vi "UHR-Fleezers Control (host) -Leonardo 04-2018 V3.vi"(0 "Tab Control":T5(tab)=enum."Trap Control (RF)") -> ()   [LabVIEW 2013] (continued)
      event "Phase adj. (AI1)", "+ phase (AI1)", "- phase (AI1)": Value Change {
        n481 = event-data() -> ()  [unwired: 7 out]
        n482 = Negate(x="Phase adj. (AI1)") -> (-x=w846:i16)
        n483 = Select(t=w846, s="- phase (AI1)", f="Phase adj. (AI1)") -> (s? t:f=w845:i16)
        n484 = xnode "Read/Write Control"("FPGA VI Reference In"=w849, "error in"=w848, "Phase count adjustment"=w845) -> ("FPGA VI Reference Out"=w844:T20, "error out"=w843:errorcluster)
        n485 = Or(x="- phase (AI1)", y="+ phase (AI1)") -> (x .or. y?=w840:bool)
        n486 = xnode "Read/Write Control"("FPGA VI Reference In"=w844, "error in"=w843, "+ phase"=w840) -> ("error out"=w839:errorcluster)  [unwired: 1 out]
      }
      event "Signals to Plot": Double Click {
        w852 = u32 9868950 ("Color Box")
        n487 = event-data() -> ("Row"=w854:i32)  [unwired: 9 out]
        n488 = property on="All Signals" class="WFChart (strict)"("Active Plot"=w854) -> (error out=w865:errorcluster)  [unwired: 2 in, 1 out]
        n489 = property on="All Signals" class="WFChart (strict)" props=["Plot", "Visible?", "Plot", "Plot Color"](error in=w865) -> (error out=w864:errorcluster, "Plot.Visible?"=w863:bool)  [unwired: 1 in, 2 out]
        n490 = Select(t=FALSE ("Plot.Visible"), s=w863, f=TRUE ("Plot.Visible")) -> (s? t:f=w858:bool)
        n491 = property on="All Signals" class="WFChart (strict)"(error in=w864, "Plot.Visible?"=w858) -> (error out=w860:errorcluster)  [unwired: 1 in, 1 out]
        n492 = property on="All Signals" class="WFChart (strict)"(error in=w860) -> (error out=w855:errorcluster, "Plot.Plot Color"=w859:u32)  [unwired: 1 in, 1 out]
        n493 = property on="Signals to Plot" class="LstBox (strict)"(error in=w855, "Active Row"=w854) -> (error out=w853:errorcluster)  [unwired: 1 in, 1 out]
        n494 = Select(t=w859, s=w858, f=u32 0) -> (s? t:f=w856:u32)
        n495 = property on="Signals to Plot" class="LstBox (strict)"(error in=w853, "CellFontColor"=w856, "SelColor"=w852, "CellBG"=w852, "CellFontSize"=u32 20 ("Active Row:Cell Font:Size"), "CellFontBold"=TRUE ("Active Row:Cell Font:Bold")) -> ()  [unwired: 1 in, 2 out]
      }
      event "Dynamic Force FB": Value Change {
        n496 = event-data() -> ()  [unwired: 7 out]
        n497 = xnode "Read/Write Control"("FPGA VI Reference In"=w867, "Dynamic Force FB (Ronen)"="Dynamic Force FB") -> ()  [unwired: 1 in, 2 out]
      }
      event "BD 1 Frequency 1 (MHz)", "BD 1 Frequency 2 (MHz)", "BD 1 Frequency 3 (MHz)", "BD 2 Frequency 1 (MHz)", "BD 2 Frequency 2 (MHz)", "BD 2 Frequency 3 (MHz)", "Trap Delta (MHz)": Value Change {
        # "anytime one of the frequencies is changed, write it to the RF board UNLESS Set 2 is being oscillated. The oscillation\nscript writes the frequencies to the RF board."
        n498 = event-data() -> ("CtlRef"=w870:refnum<vi>)  [unwired: 6 out]
        n499 = control-ref of="Trap Delta (MHz)"() -> (w869:refnum<vi>)
        n500 = Equal?(x=w869, y=w870) -> (x = y?=w868:bool)
        n501 = case shown="False" "Oscillate Set 2" {
          tunnel: w873 -> [w894 _]
          tunnel: [w893 w906] -> w872
          tunnel: w871 -> [w892 w906]
          tunnel: w868 -> [w879 _]
          frame False {
            n502 = case shown="False" "Symmetric manual \ntrap motion" {
              tunnel: ["T2 for asymmetric\n(MHz)" w905] -> w880
              tunnel: "Trap Delta (MHz)" -> [w899 w904]
              tunnel: [w898 w901] -> w876
              frame False {
                n503 = Subtract(x="T2 for asymmetric\n(MHz)", y=w899) -> (x-y=w898:dbl)
              }
              frame True {
                n504 = Divide(x=w904, y=2) -> (x/y=w902:dbl)
                n505 = Subtract(x="Middle freq for \nsymmetric (MHz)", y=w902) -> (x-y=w901:dbl)
                n506 = Add(x="Middle freq for \nsymmetric (MHz)", y=w902) -> (x+y=w905:dbl)
              }
            }
            n507 = local read "BD 1 Frequency 2 (MHz)"() -> (w881:dbl)
            n508 = local write "BD 1 Frequency 1 (MHz)"(w876) -> ()
            n509 = Select(t=w880, s=w879, f=w881) -> (s? t:f=w878:dbl)
            n510 = local read "Y RF Frequency Limits (MHz)"() -> (w882:T16)
            n511 = local read "X RF Frequency Limits (MHz)"() -> (w883:T16)
            n512 = local read "BD 1 Frequency 3 (MHz)"() -> (w895:dbl)
            n513 = local write "BD 1 Frequency 2 (MHz)"(w878) -> ()
            n514 = local read "BD 2 Frequency 1 (MHz)"() -> (w886:dbl)
            n515 = local read "BD 2 Frequency 2 (MHz)"() -> (w885:dbl)
            n516 = local read "BD 2 Frequency 3 (MHz)"() -> (w896:dbl)
            n517 = call "set RF board frequency - interlace.vi"("Board 2 Frequency Limits"=w882, "Board 1 Frequency Limits"=w883, "error in"=w892, "FPGA VI Reference In"=w894, "Board 2 Frequency 3 (MHz)"=w896, "Board 1 Frequency 3 (MHz)"=w895, "Board 2 Frequency 2 (MHz)"=w885, "Board 2 Frequency 1 (MHz)"=w886, "Board 1 Frequency 2 (MHz)"=w878, "Board 1 Frequency 1  (MHz)"=w876) -> ("error out"=w893:errorcluster)  [unwired: 1 out]
            n518 = Subtract(x=w886, y=w885) -> (x-y=w890:dbl)
            n519 = Subtract(x=w878, y=w876) -> (x-y=w891:dbl)
            n520 = Square(x=w890) -> (x^2=w888:dbl)
            n521 = Square(x=w891) -> (x^2=w889:dbl)
            n522 = Add(x=w889, y=w888) -> (x+y=w887:dbl)
            n523 = Square Root(x=w887) -> (sqrt(x)=w884:dbl)
            n524 = local write "Trap Delta (MHz)"(w884) -> ()
            n525 = property on="Initial delta (MHz)" class="DigNum (strict)"("Val(Sgnl)"=w884) -> ()  [unwired: 2 in, 2 out]
          }
          frame True {
          }
        }
      }
      event "Round T1 X": Value Change {
        n526 = event-data() -> ()  [unwired: 7 out]
        n527 = local read "BD 1 Frequency 1 (MHz)"() -> (w909:dbl)
        n528 = Round To Nearest(number=w909) -> (nearest integer value=w908:dbl)
        n529 = property on="BD 1 Frequency 1 (MHz)" class="DigNum (strict)"("Val(Sgnl)"=w908) -> ()  [unwired: 2 in, 2 out]
      }
      event "Round T2 X": Value Change {
        n530 = event-data() -> ()  [unwired: 7 out]
        n531 = local read "BD 1 Frequency 2 (MHz)"() -> (w911:dbl)
        n532 = Round To Nearest(number=w911) -> (nearest integer value=w910:dbl)
        n533 = property on="BD 1 Frequency 2 (MHz)" class="DigNum (strict)"("Val(Sgnl)"=w910) -> ()  [unwired: 2 in, 2 out]
      }
      event "Stop All": Value Change {
        n534 = event-data() -> ()  [unwired: 7 out]
        n535 = call "hamilton_controller.vi"("action"=T21."DISCONNECT") -> ()  [unwired: 10 in, 1 out]
        n536 = local read "Stop All"() -> (w914:bool)
      }
      event "Delayed Interlace Start": Value Change {
        n537 = event-data() -> ()  [unwired: 7 out]
        n538 = flat-sequence {
          frame #0 {
            n539 = Multiply(x="Delay to Interlace (s)", y=1000.0) -> (x*y=w917:dbl)
            n540 = Wait (ms)(milliseconds to wait=w917) -> ()  [unwired: 1 out]
          }
          frame #1 {
            n541 = property on="Green laser mode" class="RadioBtnsControl (strict)"("Val(Sgnl)"=enum32{"Laser ON", "Laser OFF", "Interlace"}."Interlace" ("Value (Signaling)")) -> ()  [unwired: 2 in, 2 out]
          }
        }
      }
      event "BD 1 Amplitude 1 (%)", "BD 1 Amplitude 2 (%)", "BD 1 Amplitude 3 (%)", "BD 2 Amplitude 1 (%)", "BD 2 Amplitude 2 (%)", "BD 2 Amplitude 3 (%)", "Trap 1 ON", "Trap 2 ON", "Trap 3 ON", "Feedback On/Off", "All FB On/Off": Value Change {
        w941 = i16 1 ("f")
        n542 = event-data() -> ()  [unwired: 7 out]
        n543 = local write "Trap 1 (ON/OFF)"("Trap 1 ON") -> ()
        n544 = local write "Trap 2 (ON/OFF)"("Trap 2 ON") -> ()
        n545 = Boolean To (0,1)(Boolean="Trap 3 ON") -> (0, 1=w942:i16)
        n546 = Boolean To (0,1)(Boolean="Trap 1 ON") -> (0, 1=w943:i16)
        n547 = Boolean To (0,1)(Boolean="Trap 2 ON") -> (0, 1=w944:i16)
        n548 = Select(t=w944, s="Trap ON/OFF X or Y Amp?", f=w941) -> (s? t:f=w939:i16)
        n549 = Select(t=w943, s="Trap ON/OFF X or Y Amp?", f=w941) -> (s? t:f=w940:i16)
        n550 = Select(t=w942, s="Trap ON/OFF X or Y Amp?", f=w941) -> (s? t:f=w938:i16)
        n551 = Select(t=w941, s="Trap ON/OFF X or Y Amp?", f=w944) -> (s? t:f=w936:i16)
        n552 = Select(t=w941, s="Trap ON/OFF X or Y Amp?", f=w943) -> (s? t:f=w937:i16)
        n553 = Select(t=w941, s="Trap ON/OFF X or Y Amp?", f=w942) -> (s? t:f=w935:i16)
        n554 = And(x="All FB On/Off", y="Feedback On/Off") -> (x .and. y?=w933:cluster{"Set 1":bool, "Set 2":bool})
        n555 = local read "BD 1 Amplitude 1 (%)"() -> (w953:dbl)
        n556 = local read "BD 1 Amplitude 2 (%)"() -> (w952:dbl)
        n557 = local read "BD 1 Amplitude 3 (%)"() -> (w951:dbl)
        n558 = Unbundle By Name(w933) -> ("Set 1"=w929:bool, "Set 2"=w926:bool)
        n559 = local read "Y RF Amplitude Limits (%)"() -> (w922:T16)
        n560 = local read "X RF Amplitude Limits (%)"() -> (w923:T16)
        n561 = local read "BD 2 Amplitude 1 (%)"() -> (w954:dbl)
        n562 = local read "BD 2 Amplitude 2 (%)"() -> (w955:dbl)
        n563 = local read "BD 2 Amplitude 3 (%)"() -> (w956:dbl)
        n564 = And(x="Trap 2 ON", y=w926) -> (x .and. y?=w924:bool)
        n565 = And(x="Trap 1 ON", y=w929) -> (x .and. y?=w927:bool)
        n566 = Multiply(x=w940, y=w953) -> (x*y=w948:dbl)
        n567 = Multiply(x=w952, y=w939) -> (x*y=w946:dbl)
        n568 = Multiply(x=w951, y=w938) -> (x*y=w947:dbl)
        n569 = Multiply(x=w954, y=w937) -> (x*y=w957:dbl)
        n570 = Multiply(x=w955, y=w936) -> (x*y=w958:dbl)
        n571 = Multiply(x=w956, y=w935) -> (x*y=w959:dbl)
        n572 = call "set RF board amplitude - interlace.vi"("Board 2 Amplitude Limits"=w922, "Board 1 Amplitude Limits"=w923, "error in"=w949, "FPGA VI Reference In"=w950, "Board 2 Amplitude 3 (%)"=w959, "Board 1 Amplitude 3 (%)"=w947, "Board 2 Amplitude 2 (%)"=w958, "Board 2 Amplitude 1 (%)"=w957, "Board 1 Amplitude 2 (%)"=w946, "Board 1 Amplitude 1 (%)"=w948) -> ("error out"=w931:errorcluster, "FPGA VI Reference Out"=w932:T20)
        n573 = xnode "Read/Write Control"("FPGA VI Reference In"=w932, "error in"=w931, "FB On/Off Set 1"=w927, "FB On/Off Set 2"=w924) -> ("error out"=w930:errorcluster)  [unwired: 1 out]
        n574 = case shown="True" "All FB On/Off" {
          frame False {
          }
          frame True {
            n575 = local write "Feedback overload"(FALSE) -> ()
          }
        }
      }
      event "Load parameters": Value Change {
        n576 = event-data() -> ()  [unwired: 7 out]
        n577 = property on="Saved AOD Raster Scan Parameter Sets" class="Arr (strict)"() -> ("Index Values"=w971:u32[])  [unwired: 2 in, 2 out]
        n578 = Index Array(array=w971, index=0) -> (element=w968:u32)
        n579 = local write "Load parameters"(FALSE ("Load parameters")) -> ()
        n580 = Index Array(array="Saved AOD Raster Scan Parameter Sets", index=w968) -> (element=w967:T31)
        n581 = Unbundle By Name(w967) -> ("Scan Range AOD (nm) 2"=w966:dbl, "Step Size AOD (nm) 2"=w965:dbl, "Scan Speed AOD (nm/s) 2"=w964:dbl, "Number of scans (AOD) 2"=w963:u16)
        n582 = flat-sequence {
          tunnel: w966 -> [w974]
          tunnel: w965 -> [w973]
          tunnel: w964 -> [w972]
          tunnel: w963 -> [w975]
          frame #0 {
            n583 = local write "Scan Speed (nm/s)"(w972) -> ()
            n584 = local write "Scan Range (nm)"(w974) -> ()
            n585 = local write "Step Size (nm)"(w973) -> ()
          }
          frame #1 {
            n586 = property on="Number of F/B Scans (AOD)" class="DigNum (strict)"("Val(Sgnl)"=w975) -> ()  [unwired: 2 in, 2 out]
          }
        }
      }
      event "Trap 1 (ON/OFF)", "Trap 2 (ON/OFF)": Value Change {
        n587 = event-data() -> ()  [unwired: 7 out]
        n588 = property on="Trap 2 ON" class="Bool (strict)"("Val(Sgnl)"="Trap 2 (ON/OFF)") -> ()  [unwired: 2 in, 2 out]
        n589 = property on="Trap 1 ON" class="Bool (strict)"("Val(Sgnl)"="Trap 1 (ON/OFF)") -> ()  [unwired: 2 in, 2 out]
      }
      event "DIO count 1 (ticks)", "DIO count 2 (ticks)", "DIO count 3 (ticks)", "Interlace", "Number Interlace Sets", "Not-Interlacing Set": Value Change {
        n590 = event-data() -> ()  [unwired: 7 out]
        n591 = local read "DIO count 3 (ticks)"() -> (w988:u32)
        n592 = local read "DIO count 1 (ticks)"() -> (w990:u32)
        n593 = local read "DIO count 2 (ticks)"() -> (w989:u32)
        n594 = To Unsigned Byte Integer(number="Not-Interlacing Set") -> (unsigned 8bit integer=w979:u8)
        n595 = Add(x=w979, y=u8 1) -> (x+y=w983:u8)
        n596 = xnode "Read/Write Control"("FPGA VI Reference In"=w994, "error in"=w992, "DIO count 1 (ticks)"=w990, "DIO count 2 (ticks)"=w989, "DIO count 3 (ticks)"=w988, "Interlace ON/OFF"="Interlace", "Number Interlace Cycles"="Number Interlace Sets", "Interlace Off Parameters"=w983) -> ("error out"=w993:errorcluster)  [unwired: 1 out]
        n597 = Build Array(w990, w989, w988) -> (w981:u32[])
        n598 = Split 1D Array(array=w981, index="Number Interlace Sets") -> (first subarray=w991:u32[])  [unwired: 1 out]
        n599 = Index Array(array=w981, index=w979) -> (element=w980:u32)
        n600 = Add Array Elements(numeric array=w991) -> (sum=w985:u32)
        n601 = Select(t=w985, s="Interlace", f=w980) -> (s? t:f=→"Total Counts (ticks)":u32)
      }
      event "Reset Feedback": Value Change {
        n602 = event-data() -> ()  [unwired: 7 out]
        n603 = Unbundle By Name("Reset Feedback") -> ("Set 1"=w998:bool, "Set 2"=w997:bool)
        n604 = xnode "Read/Write Control"("FPGA VI Reference In"=w1000, "error in"=w995, "FB Reset Set 1"=w998, "FB Reset Set 2"=w997) -> ("error out"=w996:errorcluster)  [unwired: 1 out]
      }
      event "PID gains": Value Change {
        n605 = event-data() -> ()  [unwired: 7 out]
        n606 = local read "PID gains"() -> (w1001:T10)
        n607 = xnode "Read/Write Control"("FPGA VI Reference In"=w1004, "error in"=w1002, "FB Gains"=w1001) -> ("error out"=w1003:errorcluster)  [unwired: 1 out]
      }
      event "AI2 to Setpoint", "Trap Intensity\nSetpoints (V)": Value Change {
        n608 = event-data() -> ()  [unwired: 7 out]
        n609 = xnode "Read/Write Control"("FPGA VI Reference In"=w1009, "error in"=w1005) -> ("FPGA VI Reference Out"=w1008:T20, "error out"=w1007:errorcluster, "AI2 Y Sum Set 1"=w1016:i16, "AI2 Y Sum Set 2"=w1015:i16)
        n610 = Cluster To Array(cluster="AI2 to Setpoint") -> (array=w1019:bool[])
        n611 = local read "AI2 (V)"() -> (w1017:cluster{"Set 1":dbl, "Set 2":dbl})
        n612 = Or Array Elements(Boolean array=w1019) -> (logical OR=w1020:bool)
        n613 = Bundle By Name(cluster=w1017, "Set 1"=w1016, "Set 2"=w1015) -> (w1014:cluster{"Set 1":dbl, "Set 2":dbl})
        n614 = Divide(x=w1014, y=3276.7) -> (x/y=w1013:cluster{"Set 1":dbl, "Set 2":dbl})
        "AI2 (V)" <- w1013
        n615 = case shown="False" w1020 {
          tunnel: [w1023 w1040] -> w1012
          tunnel: "AI2 to Setpoint" -> [_ w1036]
          tunnel: "Trap Intensity\nSetpoints (V)" -> [w1024 w1039]
          tunnel: w1013 -> [_ w1033]
          frame False {
            n616 = Multiply(x=3276.7, y=w1024) -> (x*y=w1025:cluster{"Set 1":dbl, "Set 2":dbl})
            n617 = To Word Integer(number=w1025) -> (16bit integer=w1023:cluster{"Set 1":i16, "Set 2":i16})
          }
          frame True {
            n618 = Unbundle By Name(w1033) -> ("Set 1"=w1032:dbl, "Set 2"=w1031:dbl)
            n619 = Unbundle By Name(w1039) -> ("Set 1"=w1038:dbl, "Set 2"=w1037:dbl)
            n620 = Unbundle By Name(w1036) -> ("Set 1"=w1035:bool, "Set 2"=w1034:bool)
            n621 = Select(t=w1032, s=w1035, f=w1038) -> (s? t:f=w1030:dbl)
            n622 = Select(t=w1031, s=w1034, f=w1037) -> (s? t:f=w1029:dbl)
            n623 = Bundle By Name(cluster=w1039, "Set 1"=w1030, "Set 2"=w1029) -> (w1027:cluster{"Set 1":dbl, "Set 2":dbl})
            n624 = local write "Trap Intensity\nSetpoints (V)"(w1027) -> ()
            n625 = Multiply(x=3276.7, y=w1027) -> (x*y=w1028:cluster{"Set 1":dbl, "Set 2":dbl})
            n626 = To Word Integer(number=w1028) -> (16bit integer=w1040:cluster{"Set 1":i16, "Set 2":i16})
          }
        }
        n627 = Unbundle By Name(w1012) -> ("Set 1"=w1011:i16, "Set 2"=w1010:i16)
        n628 = xnode "Read/Write Control"("FPGA VI Reference In"=w1008, "error in"=w1007, "FB Setpoint Set 1"=w1011, "FB Setpoint Set 2"=w1010) -> ("error out"=w1006:errorcluster)  [unwired: 1 out]
      }
      event "Invert GI": Value Change {
        n629 = event-data() -> ()  [unwired: 7 out]
        n630 = xnode "Read/Write Control"("FPGA VI Reference In"=w1045, "error in"=w1043, "Invert GI"="Invert GI", "Invert GI 2"="Invert GI") -> ("error out"=w1044:errorcluster)  [unwired: 1 out]
      }
      event "Green FB Setpoint (mV)", "Green FB Gains", "Green FB On/Off", "Current When FB OFF (%)", "Green int current ON count adj": Value Change {
        n631 = event-data() -> ()  [unwired: 7 out]
        n632 = local read "Green FB Setpoint (mV)"() -> (w1052:dbl)
        n633 = local read "Current When FB OFF (%)"() -> (w1055:dbl)
        n634 = Multiply(x=w1052, y=3.2767) -> (x*y=w1051:dbl)
        n635 = Multiply(x=w1055, y=655.35) -> (x*y=w1056:dbl)
        n636 = To Unsigned Word Integer(number=w1056) -> (unsigned 16bit integer=w1054:u16)
        n637 = local read "Green int current ON count adj"() -> (w1059:u32)
        n638 = local read "Green FB Gains"() -> (w1058:T10)
        n639 = local read "Green Laser ON/Interlacing"() -> (w1049:bool)
        n640 = local read "Green laser mode"() -> (w1048:enum32{"Laser ON", "Laser OFF", "Interlace"})
        n641 = local read "Green FB On/Off"() -> (w1060:bool)
        n642 = Equal?(x=w1048, y=enum32{"Laser ON", "Laser OFF", "Interlace"}."Interlace") -> (x = y?=w1046:bool)
        n643 = Compound Arithmetic op=AND(w1046, w1060, w1049) -> (w1050:bool)
        n644 = xnode "Read/Write Control"("FPGA VI Reference In"=w1063, "error in"=w1062, "Green FB Setpoint"=w1051, "Green FB On/Off"=w1050, "Current Out"=w1054, "Green int current ON count adj"=w1059, "Green FB Gains"=w1058) -> ("error out"=w1061:errorcluster)  [unwired: 1 out]
      }
      event "Green laser mode", "Green Laser ON/Interlacing": Value Change {
        n645 = event-data() -> ()  [unwired: 7 out]
        n646 = case shown="True" "Green Laser ON/Interlacing" {
          tunnel: "Green laser mode" -> [_ w1077]
          tunnel: [enum32{"Laser ON", "Laser OFF", "Interlace"}."Laser OFF" ("Green laser mode") w1077] -> w1065
          tunnel: [FALSE w1073] -> w1064
          frame False {
          }
          frame True {
            n647 = local read "Green FB On/Off"() -> (w1074:bool)
            n648 = Equal?(x=w1077, y=enum32{"Laser ON", "Laser OFF", "Interlace"}."Interlace") -> (x = y?=w1075:bool)
            n649 = And(x=w1075, y=w1074) -> (x .and. y?=w1073:bool)
          }
        }
        n650 = xnode "Read/Write Control"("FPGA VI Reference In"=w1070, "error in"=w1068, "Operating Mode"=w1065, "Operating Mode 2"=w1065, "Green FB On/Off"=w1064) -> ("error out"=w1069:errorcluster)  [unwired: 1 out]
      }
      event "- phase (APD 1 Gate)", "+ phase (APD 1 Gate)": Value Change {
        n651 = event-data() -> ()  [unwired: 7 out]
        n652 = local read "Phase Adj. (APD 1 Gate)"() -> (w1078:i16)
        n653 = Negate(x=w1078) -> (-x=w1086:i16)
        n654 = Select(t=w1086, s="- phase (APD 1 Gate)", f=w1078) -> (s? t:f=w1085:i16)
        n655 = Or(x="- phase (APD 1 Gate)", y="+ phase (APD 1 Gate)") -> (x .or. y?=w1081:bool)
        n656 = xnode "Read/Write Control"("FPGA VI Reference In"=w1088, "error in"=w1087, "Phase count adjustment (APD 1 Gate)"=w1085) -> ("FPGA VI Reference Out"=w1083:T20, "error out"=w1084:errorcluster)
        n657 = xnode "Read/Write Control"("FPGA VI Reference In"=w1083, "error in"=w1084, "+ phase (APD 1 Gate)"=w1081) -> ("error out"=w1082:errorcluster)  [unwired: 1 out]
      }
      event "+ phase (APD 2 Gate)", "- phase (APD 2 Gate)": Value Change {
        n658 = event-data() -> ()  [unwired: 7 out]
        n659 = local read "Phase Adj. (APD 2 Gate)"() -> (w1089:i16)
        n660 = Negate(x=w1089) -> (-x=w1097:i16)
        n661 = Select(t=w1097, s="- phase (APD 2 Gate)", f=w1089) -> (s? t:f=w1096:i16)
        n662 = Or(x="- phase (APD 2 Gate)", y="+ phase (APD 2 Gate)") -> (x .or. y?=w1092:bool)
        n663 = xnode "Read/Write Control"("FPGA VI Reference In"=w1099, "error in"=w1098, "Phase count adjustment (APD 2 Gate)"=w1096) -> ("FPGA VI Reference Out"=w1094:T20, "error out"=w1095:errorcluster)
        n664 = xnode "Read/Write Control"("FPGA VI Reference In"=w1094, "error in"=w1095, "+ phase (APD 2 Gate)"=w1092) -> ("error out"=w1093:errorcluster)  [unwired: 1 out]
      }
      event "Phase Adj. (APD Acq)", "+ phase (APD Acq)", "- phase (APD Acq)": Value Change {
        n665 = event-data() -> ()  [unwired: 7 out]
        n666 = local read "Phase Adj. (APD Acq)"() -> (w1102:i16)
        n667 = Negate(x=w1102) -> (-x=w1108:i16)
        n668 = Select(t=w1108, s="+ phase (APD Acq)", f=w1102) -> (s? t:f=w1107:i16)
        n669 = Or(x="+ phase (APD Acq)", y="- phase (APD Acq)") -> (x .or. y?=w1103:bool)
        n670 = xnode "Read/Write Control"("FPGA VI Reference In"=w1110, "error in"=w1109, "Phase Count Adjustment (APD Acq)"=w1107) -> ("FPGA VI Reference Out"=w1105:T20, "error out"=w1106:errorcluster)
        n671 = xnode "Read/Write Control"("FPGA VI Reference In"=w1105, "error in"=w1106, "+ phase (APD Acq)"=w1103) -> ("error out"=w1104:errorcluster)  [unwired: 1 out]
      }
      event "Phase adj. (GI)", "+ phase (GI)", "- phase (GI)": Value Change {
        n672 = event-data() -> ()  [unwired: 7 out]
        n673 = Negate(x="Phase adj. (GI)") -> (-x=w1119:i16)
        n674 = Select(t=w1119, s="+ phase (GI)", f="Phase adj. (GI)") -> (s? t:f=w1118:i16)
        n675 = Or(x="+ phase (GI)", y="- phase (GI)") -> (x .or. y?=w1114:bool)
        n676 = xnode "Read/Write Control"("FPGA VI Reference In"=w1121, "error in"=w1120, "Phase count adjustment (GI)"=w1118) -> ("FPGA VI Reference Out"=w1116:T20, "error out"=w1117:errorcluster)
        n677 = xnode "Read/Write Control"("FPGA VI Reference In"=w1116, "error in"=w1117, "+ phase (GI)"=w1114) -> ("error out"=w1115:errorcluster)  [unwired: 1 out]
      }
      event "Phase adj. (GI) 2", "+ phase (GI) 2", "- phase (GI) 2": Value Change {
        n678 = event-data() -> ()  [unwired: 7 out]
        n679 = Negate(x="Phase adj. (GI) 2") -> (-x=w1130:i16)
        n680 = Select(t=w1130, s="+ phase (GI) 2", f="Phase adj. (GI) 2") -> (s? t:f=w1129:i16)
        n681 = Or(x="+ phase (GI) 2", y="- phase (GI) 2") -> (x .or. y?=w1125:bool)
        n682 = xnode "Read/Write Control"("FPGA VI Reference In"=w1132, "error in"=w1131, "Phase count adjustment (GI) 2"=w1129) -> ("FPGA VI Reference Out"=w1127:T20, "error out"=w1128:errorcluster)
        n683 = xnode "Read/Write Control"("FPGA VI Reference In"=w1127, "error in"=w1128, "+ phase (GI) 2"=w1125) -> ("error out"=w1126:errorcluster)  [unwired: 1 out]
      }
      event "Phase adj. (Green FB)", "- phase (Green FB)", "+ phase (Green FB)": Value Change {
        n684 = event-data() -> ()  [unwired: 7 out]
        n685 = Negate(x="Phase adj. (Green FB)") -> (-x=w1141:i16)
        n686 = Select(t=w1141, s="+ phase (Green FB)", f="Phase adj. (Green FB)") -> (s? t:f=w1140:i16)
        n687 = Or(x="+ phase (Green FB)", y="- phase (Green FB)") -> (x .or. y?=w1136:bool)
        n688 = xnode "Read/Write Control"("FPGA VI Reference In"=w1143, "error in"=w1142, "Phase count adjustment (Green FB)"=w1140) -> ("FPGA VI Reference Out"=w1138:T20, "error out"=w1139:errorcluster)
        n689 = xnode "Read/Write Control"("FPGA VI Reference In"=w1138, "error in"=w1139, "+ phase (Green FB)"=w1136) -> ("error out"=w1137:errorcluster)  [unwired: 1 out]
      }
      event "Invert APD Gate", "APD Gate ON Count", "APD Gate OFF Count", "APD Gate", "APD Integration Time (s)", "APD 1 AO Mult.", "APD 2 AO Mult.": Value Change {
        n690 = event-data() -> ()  [unwired: 7 out]
        n691 = local read "APD Integration Time (s)"() -> (w1144:dbl)
        n692 = local read "APD Gate ON Count"() -> (w1157:u32)
        n693 = local read "APD Gate OFF Count"() -> (w1156:u32)
        n694 = local read "Invert APD Gate"() -> (w1158:bool)
        n695 = local read "APD Gate"() -> (w1155:enum32{"ON", "OFF", "Interlace"})
        n696 = Multiply(x=w1144, y=40000000.0) -> (x*y=w1153:dbl)
        n697 = Reciprocal(x=w1144) -> (1/x=→"APD Acq Rate (Hz)":dbl)
        n698 = To Unsigned Long Integer(number=w1153) -> (unsigned 32bit integer=w1152:u32)
        n699 = local read "DMA Update Period (s)"() -> (w1145:dbl)
        n700 = Divide(x=w1145, y=w1144) -> (x/y=w1148:dbl)
        n701 = local read "APD 1 AO Mult."() -> (w1150:i16)
        n702 = local read "APD 2 AO Mult."() -> (w1149:i16)
        n703 = Multiply(x=2.0, y=w1148) -> (x*y=w1147:dbl)
        n704 = local write "APD Samples/FIFO Acq."(w1148) -> ()
        n705 = local write "APD Elements/DMA read"(w1147) -> ()
        n706 = xnode "Read/Write Control"("FPGA VI Reference In"=w1161, "error in"=w1160, "Invert APD Gate"=w1158, "APD Gate ON Count"=w1157, "APD Gate OFF Count"=w1156, "APD Acq Rate Count"=w1152, "APD Gate Operating Mode"=w1155, "APD 1 AO scale factor"=w1150, "APD 2 AO scale factor"=w1149) -> ("error out"=w1159:errorcluster)  [unwired: 1 out]
      }
      event "GI Frequency, ON count", "Green FB Count", "GI Frequency, OFF count": Value Change {
        n707 = event-data() -> ()  [unwired: 7 out]
        n708 = xnode "Read/Write Control"("FPGA VI Reference In"=w1167, "error in"=w1165, "Green interlace ON count"="GI Frequency, ON count", "Green interlace OFF count"="GI Frequency, OFF count", "Green interlace ON count 2"="GI Frequency, ON count", "Green interlace OFF count 2"="GI Frequency, OFF count", "Green FB Count"="Green FB Count") -> ("error out"=w1166:errorcluster)  [unwired: 1 out]
      }
      event "Number of F/B Scans (AOD)", "Scan Speed (nm/s)", "Scan BD", "Initial delta (MHz)", "Step Size (nm)", "Scan Range (nm)": Value Change {
        w1229 = 123.0  # AOM cal (nm/MHz)
        n709 = event-data() -> ()  [unwired: 7 out]
        n710 = local read "BD 1 Frequency 1 (MHz)"() -> (w1212:dbl)
        n711 = local read "AOM X Cal (nm/MHz)"() -> (w1204:dbl)
        n712 = local read "X RF Frequency Limits (MHz)"() -> (w1216:T16)
        n713 = local read "Y RF Frequency Limits (MHz)"() -> (w1213:T16)
        n714 = local read "BD 2 Frequency 1 (MHz)"() -> (w1218:dbl)
        n715 = Negate(x="Scan Range (nm)") -> (-x=w1182:dbl)
        n716 = Divide(x=w1182, y=w1204) -> (x/y=w1186:dbl)
        n717 = Select(t=w1216, s="Scan BD", f=w1213) -> (s? t:f=w1215:T16)
        n718 = Select(t=w1212, s="Scan BD", f=w1218) -> (s? t:f=w1217:dbl)
        n719 = Unbundle By Name(w1215) -> ("Maximum"=w1224:dbl, "Minimum"=w1223:dbl)
        n720 = Add(x=w1186, y=w1217) -> (x+y=w1221:dbl)
        n721 = Divide(x=w1182, y="Step Size (nm)") -> (x/y=w1201:dbl)
        n722 = Divide(x="Step Size (nm)", y=w1204) -> (x/y=w1210:dbl)
        n723 = Absolute Value(x=w1201) -> (abs(x)=w1185:dbl)
        n724 = Sign(1:w1182) -> (0:w1183:dbl)
        n725 = In Range and Coerce(upper limit=w1224, x=w1221, lower limit=w1223) -> (coerced(x)=w1220:dbl, In Range?=w1222:bool)
        n726 = To Unsigned Quad Integer(1:w1185) -> (0:w1200:u64)
        "Scan steps (AOD)" <- w1200
        n727 = call "IR AOM freq to word.vi"("Frequency In (MHz)"=w1210) -> ("Frequency Word Out (double)"=w1207:dbl)
        n728 = Multiply(x=w1183, y=w1207) -> (x*y=w1184:dbl)
        n729 = Subtract(x=w1221, y=w1220) -> (x-y=w1219:dbl)
        n730 = To Quad Integer(1:w1184) -> (0:w1206:i64)
        "Incr. int (AOD)" <- w1206
        n731 = Subtract(x=w1186, y=w1219) -> (x-y=w1205:dbl)
        "Scan Range (MHz)" <- w1205
        n732 = Select(t=w1186, s=w1222, f=w1205) -> (s? t:f=w1225:dbl)
        n733 = Multiply(x=w1205, y=w1204) -> (x*y=w1203:dbl)
        n734 = Decrement(x=w1200) -> (x-1=w1253:u64)
        n735 = Negate(x=w1203) -> (-x=w1199:dbl)
        n736 = local write "Scan Range (nm)"(w1199) -> ()
        n737 = Divide(x=w1225, y=w1253) -> (x/y=w1209:dbl)
        "Scan Increment (MHz)" <- w1209
        n738 = call "IR AOM freq to word.vi"("Frequency In (MHz)"=w1209) -> ("Frequency Word Out (double)"=w1208:dbl)
        n739 = Divide(x="Step Size (nm)", y="Scan Speed (nm/s)") -> (x/y=w1196:dbl)
        n740 = To Quad Integer(1:w1208) -> ()  [unwired: 1 out]
        n741 = local read "Number Interlace Sets"() -> (w1180:u8)
        n742 = local read "AI Count (ticks)"() -> (w1181:u32)
        n743 = local read "Total Counts (ticks)"() -> (w1179:u32)
        n744 = local read "# Samples/trap"() -> (w1211:u32)
        n745 = Multiply(x=w1181, y=w1180) -> (x*y=w1178:u32)
        n746 = Divide(x=w1179, y=w1178) -> (x/y=w1177:dbl)
        n747 = Select(t=w1212, s="Scan BD", f=w1218) -> (s? t:f=w1250:dbl)
        "Initial freq. (MHz)" <- w1250
        n748 = Add(x=w1225, y=w1250) -> (x+y=→"Final freq. (MHz)":dbl)
        n749 = Divide(x=w1179, y=40000000.0) -> (x/y=w1195:dbl)
        n750 = Divide(x=w1196, y=w1195) -> (x/y=w1194:dbl)
        n751 = To Unsigned Quad Integer(1:w1194) -> (0:w1169:u64)
        n752 = Quotient & Remainder(x=w1169, y=u64 2) -> (x-y*floor(x/y)=w1173:u64)  [unwired: 1 out]
        n753 = Equal?(x=w1173, y=u64 0) -> (x = y?=w1171:bool)
        n754 = Decrement(x=w1169) -> (x-1=w1170:u64)
        n755 = Select(t=w1169, s=w1171, f=w1170) -> (s? t:f=w1168:u64)
        "Cycles/step (AOD)" <- w1168
        n756 = xnode "Read/Write Control"("FPGA VI Reference In"=w1261, "error in"=w1260, "Scan steps"=w1200, "Number of scans"="Number of F/B Scans (AOD)", "Cycles per step"=w1168, "Scan freq.  increment"=w1206, "Scan BD"="Scan BD") -> ("error out"=w1259:errorcluster)  [unwired: 1 out]
        n757 = Multiply(x=w1200, y=w1168) -> (x*y=w1254:u64)
        n758 = Multiply(x=w1254, y=u64 2) -> (x*y=w1176:u64)
        n759 = Multiply(x=w1177, y=w1176) -> (x*y=w1175:dbl)
        "Data points/scan (f/b)" <- w1175
        n760 = Multiply(x=w1175, y="Number of F/B Scans (AOD)") -> (x*y=w1257:dbl)
        "Data points/scans" <- w1257
        n761 = Divide(x=w1257, y=w1211) -> (x/y=→"N sets should be saved":dbl)
        n762 = Multiply(x=w1254, y=w1195) -> (x*y=w1193:dbl)
        "Time/Scan (s) (AOD)" <- w1193
        n763 = Select(t=w1225, s="Scan BD", f=0.0) -> (s? t:f=w1251:dbl)
        n764 = Select(t=0.0, s="Scan BD", f=w1225) -> (s? t:f=w1247:dbl)
        n765 = local read "BD 2 Frequency 2 (MHz)"() -> (w1243:dbl)
        n766 = local read "BD 1 Frequency 2 (MHz)"() -> (w1246:dbl)
        n767 = Add(x=w1247, y=w1218) -> (x+y=w1244:dbl)
        n768 = Add(x=w1212, y=w1251) -> (x+y=w1245:dbl)
        n769 = Multiply(x=w1193, y=2.0) -> (x*y=w1192:dbl)
        n770 = Multiply(x=w1192, y="Number of F/B Scans (AOD)") -> (x*y=w1189:dbl)
        n771 = Divide(x=w1189, y=60.0) -> (x/y=→"Time to Finish All (min)":dbl)
        n772 = Add(x="Trap 2 Bead Size (nm)", y="Trap 1 Bead Size (nm)") -> (x+y=w1233:dbl)
        n773 = local read "Initial delta (MHz)"() -> (w1230:dbl)
        n774 = Divide(x=w1233, y=2.0) -> (x/y=w1227:dbl)
        n775 = Subtract(x=w1244, y=w1243) -> (x-y=w1241:dbl)
        n776 = Subtract(x=w1245, y=w1246) -> (x-y=w1242:dbl)
        n777 = Square(x=w1241) -> (x^2=w1240:dbl)
        n778 = Square(x=w1242) -> (x^2=w1239:dbl)
        n779 = Add(x=w1239, y=w1240) -> (x+y=w1238:dbl)
        n780 = Square Root(x=w1238) -> (sqrt(x)=w1237:dbl)
        "Final delta (MHz)" <- w1237
        n781 = Multiply(x=w1229, y=w1237) -> (x*y=w1236:dbl)
        n782 = Multiply(x=w1230, y=w1229) -> (x*y=w1228:dbl)
        n783 = Subtract(x=w1228, y=w1227) -> (x-y=→"Initial sep (nm)":dbl)
        n784 = Subtract(x=w1236, y=w1227) -> (x-y=→"Final sep (nm)":dbl)
      }
      event "Raster Scanning...": Value Change {
        n785 = event-data() -> ("NewVal"=w1262:bool)  [unwired: 6 out]
        n786 = case shown="True" w1262 {
          frame False {
          }
          frame True {
            n787 = property on="BD 1 Frequency 1 (MHz)" class="DigNum (strict)"("Val(Sgnl)"=65.0 ("Value (Signaling)")) -> ()  [unwired: 2 in, 2 out]
          }
        }
      }
      event "Phase increment trap 1", "Swap F1 and F2", "Freq switch delay", "Amp switch delay", "Phase increment trap 2", "RF phase reset before cycles", "Phase offset method": Value Change {
        n788 = event-data() -> ()  [unwired: 7 out]
        n789 = local read "Amp switch delay"() -> (w1268:u16)
        n790 = local read "Phase increment trap 1"() -> (w1267:fxp<+/-,64,32>)
        n791 = local read "Freq switch delay"() -> (w1270:u16)
        n792 = local read "Phase increment trap 2"() -> (w1266:fxp<+/-,64,32>)
        n793 = local read "RF phase reset before cycles"() -> (w1265:bool)
        n794 = local read "Swap F1 and F2"() -> (w1269:bool)
        n795 = local read "Phase offset method"() -> (w1264:u8)
        n796 = xnode "Read/Write Control"("FPGA VI Reference In"=w1273, "error in"=w1272, "BD 1 Delay (ticks)"=w1270, "Swap F1 and F2"=w1269, "Amp switch delay"=w1268, "Phase Trap 1"=w1267, "Phase Trap 2"=w1266, "RF phase reset before cycles"=w1265, "Phase offset method"=w1264) -> ("error out"=w1271:errorcluster)  [unwired: 1 out]
      }
      event "Scan steps (MCL)", "Number of scans (MCL)", "Scan Range (V)\n(of steps)", "2D or 1D Scan", "N APD Samp/step", "Fast Scan Dir", "Continuous MCL Scanning", "Scan lines (y)": Value Change {
        w1275 = 32767.0 ("y")
        n797 = event-data() -> ()  [unwired: 7 out]
        n798 = Select(t="Scan lines (y)", s="2D or 1D Scan", f="Number of scans (MCL)") -> (s? t:f=w1280:u64)
        n799 = Decrement(x="Scan steps (MCL)") -> (x-1=w1296:u64)
        n800 = Divide(x="Scan Range (V)\n(of steps)", y=w1296) -> (x/y=w1295:dbl)
        "Desired Scan Incr (V)" <- w1295
        n801 = local read "APD Integration Time (s)"() -> (w1288:dbl)
        n802 = Multiply(x=w1295, y=w1275) -> (x*y=w1304:dbl)
        n803 = Divide(x=w1304, y=10.0) -> (x/y=w1294:dbl)
        "Desired incr (int)" <- w1294
        n804 = local read "Update Count (MCL)"() -> (w1300:u32)
        n805 = Round Toward -Infinity(1:w1294) -> (0:w1303:dbl)
        n806 = To Word Integer(number=w1303) -> (16bit integer=w1278:i16)
        "Actual Incr. int (MCL)" <- w1278
        n807 = Multiply(x=w1288, y=40000000.0) -> (x*y=w1301:dbl)
        n808 = Divide(x=w1301, y=w1300) -> (x/y=w1299:dbl)
        n809 = Multiply(x=i16 10, y=w1278) -> (x*y=w1276:i16)
        n810 = Multiply(x="N APD Samp/step", y=w1299) -> (x*y=w1298:dbl)
        "Cycles/step (MCL)" <- w1298
        n811 = Divide(x=w1276, y=w1275) -> (x/y=→"Actual MCL Inc (V)":dbl)
        n812 = Multiply(x="N APD Samp/step", y="Scan steps (MCL)") -> (x*y=w1290:dbl)
        n813 = local read "APD Samples/FIFO Acq."() -> (w1287:dbl)
        n814 = Multiply(x=w1290, y=u64 2) -> (x*y=w1289:dbl)
        "Data points/scan (f+b)" <- w1289
        n815 = Multiply(x=w1289, y=w1280) -> (x*y=w1307:dbl)
        "Data points/scans (MCL)" <- w1307
        n816 = Multiply(x=w1288, y=w1289) -> (x*y=w1281:dbl)
        "Time/f+b scan (s) (MCL)" <- w1281
        n817 = Divide(x=w1307, y=w1287) -> (x/y=→"N sets should be saved (MCL)":dbl)
        n818 = Multiply(x=w1281, y=w1280) -> (x*y=→"Total Time (s)":dbl)
        n819 = Not(x="Fast Scan Dir") -> (.not. x?=w1285:bool)
        n820 = xnode "Read/Write Control"("FPGA VI Reference In"=w1311, "error in"=w1310, "Scan steps (MCL)"="Scan steps (MCL)", "Number of scans (MCL)"=w1280, "Cycles per step (MCL)"=w1298, "Scan freq.  increment (MCL)"=w1278, "1D or 2D Scan?"="2D or 1D Scan", "MCL Scan Axis"=w1285, "Cont. Scan (MCL)"="Continuous MCL Scanning") -> ("error out"=w1309:errorcluster)  [unwired: 1 out]
      }
      event "Read Cal": Value Change {
        w1344 = 1000.0 ("y")
        w1332 = T30."big-endian, network order" ("byte order (0:big-endian, network order)")
        w1333 = -1 ("count (1)")
        n821 = event-data() -> ()  [unwired: 7 out]
        n822 = local read "Save file name"() -> (w1362:path)
        n823 = local write "Read Cal"(FALSE ("Read Cal")) -> ()
        n824 = Strip Path(path=w1362) -> (stripped path=w1361:path)  [unwired: 1 out]
        n825 = Path To String(path=w1361) -> (string=w1342:string)
        n826 = Concatenate Strings(w1342, "\\current.off" ("string")) -> (w1340:string)
        n827 = Concatenate Strings(w1342, "\\current.cal" ("string")) -> (w1359:string)
        n828 = String To Path(string=w1359) -> (path=w1358:path)
        n829 = String To Path(string=w1340) -> (path=w1339:path)
        n830 = Open/Create/Replace File(file path (use dialog)=w1358, operation (0:open)=T24."open", access (0:read/write)=enum16{"read/write", "read-only", "write-only"}."read-only") -> (refnum out=w1365:refnum<file>, error out=w1354:errorcluster)  [unwired: 1 in, 3 out]
        n831 = Deny Access(4:w1354, 7:w1365) -> (0:w1353:errorcluster, 3:w1357:refnum<file>)  [unwired: 1 out]
        n832 = Open/Create/Replace File(file path (use dialog)=w1339, operation (0:open)=T24."open", access (0:read/write)=enum16{"read/write", "read-only", "write-only"}."read-only") -> (refnum out=w1336:refnum<file>)  [unwired: 1 in, 4 out]
        n833 = Deny Access(7:w1336) -> (3:w1334:refnum<file>)  [unwired: 1 in, 2 out]
        n834 = Read from Binary File(5:0.0, 8:w1353, 9:w1332, 10:w1333, 11:w1357) -> (0:w1352:errorcluster, 2:w1350:dbl[], 3:w1355:refnum<file>)  [unwired: 2 out]
        n835 = Array To Cluster(array=w1350) -> (cluster=w1349:T32)
        n836 = Unbundle(w1349) -> ("[0]"=w1323:dbl, "[1]"=w1321:dbl, "[2]"=w1322:dbl, "[3]"=w1320:dbl, "[4]"=w1348:dbl, "[5]"=w1347:dbl)
        n837 = Close File(refnum=w1355, error in=w1352) -> (error out=→"Read cal error":errorcluster)  [unwired: 1 out]
        n838 = Multiply(x=w1347, y=w1344) -> (x*y=w1345:dbl)
        n839 = local write "T2 kappa_x (pN/nm)"(w1320) -> ()
        n840 = local write "T1 kappa_x (pN/nm)"(w1322) -> ()
        n841 = local write "T1 alpha_x (nm/V)"(w1323) -> ()
        n842 = local write "T2 alpha_x (nm/V)"(w1321) -> ()
        n843 = Read from Binary File(5:0.0, 9:w1332, 10:w1333, 11:w1334) -> (2:w1328:dbl[], 3:w1331:refnum<file>)  [unwired: 1 in, 3 out]
        n844 = Multiply(x=w1348, y=w1344) -> (x*y=w1346:dbl)
        n845 = local write "T1 offset_x (mV)"(w1346) -> ()
        n846 = local write "T2 offset_x (mV)"(w1345) -> ()
        n847 = Close File(refnum=w1331) -> ()  [unwired: 1 in, 2 out]
        n848 = Array Subset(array=w1328, index=3) -> (w1326:dbl[])  [unwired: 1 in]
        n849 = Index Array(array=w1328, index=0) -> (element=→"Offset file step size":dbl)
        n850 = Multiply(x=w1323, y=w1322) -> (x*y=w1318:dbl)
        n851 = Multiply(x=w1321, y=w1320) -> (x*y=w1319:dbl)
        n852 = Divide(x=w1319, y=w1318) -> (x/y=w1313:dbl)
        n853 = Decimate 1D Array(w1326) -> (w1316:dbl[], w1317:dbl[])  [unwired: 1 out]
        n854 = property on="B factor" class="DigNum (strict)"("Val(Sgnl)"=w1313) -> ()  [unwired: 2 in, 2 out]
        n855 = Bundle By Name(cluster="Offset Values", "Trap 1X offset"=w1316, "Trap 2X offset"=w1317) -> (w1324:T14)
        n856 = Multiply(x=w1317, y=w1313) -> (x*y=w1315:dbl[])
        n857 = Subtract(x=w1316, y=w1315) -> (x-y=w1314:dbl[])
        n858 = local write "Offset Values"(w1324) -> ()
        n859 = case shown="True" "Auto read offset\ncorrection" {
          tunnel: w1314 -> [_ w1366]
          frame False {
          }
          frame True {
            n860 = property on="Setpoint offset\nCorrection values" class="Arr (strict)"("Val(Sgnl)"=w1366) -> ()  [unwired: 2 in, 2 out]
          }
        }
      }
      event "Abort MCL Scan": Value Change {
        n861 = event-data() -> ()  [unwired: 7 out]
        n862 = local write "MCL Scanning"(FALSE ("MCL Scanning")) -> ()
        n863 = xnode "Read/Write Control"("FPGA VI Reference In"=w1371, "error in"=w1370, "Abort scan (MCL)"="Abort MCL Scan") -> ("error out"=w1369:errorcluster)  [unwired: 1 out]
      }
      event "Update Count (MCL)": Value Change {
        n864 = event-data() -> ()  [unwired: 7 out]
        n865 = xnode "Read/Write Control"("FPGA VI Reference In"=w1375, "error in"=w1374, "MCL count"="Update Count (MCL)") -> ("error out"=w1373:errorcluster)  [unwired: 1 out]
      }
      event "Phase adjust (MCL)", "+ phase (MCL)", "- phase (MCL)": Value Change {
        n866 = event-data() -> ()  [unwired: 7 out]
        n867 = Negate(x="Phase adjust (MCL)") -> (-x=w1384:i16)
        n868 = Select(t=w1384, s="- phase (MCL)", f="Phase adjust (MCL)") -> (s? t:f=w1382:i16)
        n869 = Or(x="- phase (MCL)", y="+ phase (MCL)") -> (x .or. y?=w1377:bool)
        n870 = xnode "Read/Write Control"("FPGA VI Reference In"=w1386, "error in"=w1385, "Phase count adjustment (MCL)"=w1382) -> ("FPGA VI Reference Out"=w1378:T20, "error out"=w1379:errorcluster)
        n871 = xnode "Read/Write Control"("FPGA VI Reference In"=w1378, "error in"=w1379, "+ phase (MCL)"=w1377) -> ("error out"=w1376:errorcluster)  [unwired: 1 out]
      }
      event "Abort AOD Scan": Value Change {
        n872 = event-data() -> ()  [unwired: 7 out]
        n873 = flat-sequence {
          tunnel: w1391 -> [w1398]
          tunnel: w1390 -> [w1397]
          tunnel: [w1396] -> w1388
          tunnel: [w1392] -> w1387
          tunnel: [w1411] -> w1389
          tunnel: w1388 -> [w1411]
          tunnel: w1387 -> [w1410]
          frame #0 {
            n874 = local read "Save scans"() -> (w1394:bool)
            n875 = xnode "Read/Write Control"("FPGA VI Reference In"=w1398, "error in"=w1397, "Abort scan"="Abort AOD Scan") -> ("FPGA VI Reference Out"=w1392:T20, "error out"=w1396:errorcluster)
            n876 = local write "Raster Scanning..."(FALSE) -> ()
            n877 = case shown="True" w1394 {
              frame False {
              }
              frame True {
                n878 = local write "Stop Saving"(TRUE) -> ()
              }
            }
          }
          frame #1 {
            n879 = xnode "Read/Write Control"("FPGA VI Reference In"=w1410) -> ("BD1 Frequency Out 1"=w1401:u64)  [unwired: 1 in, 2 out]
            n880 = To Double Precision Float(number=w1401) -> (double precision float=w1407:dbl)
            n881 = Multiply(x=49125000.0, y=6.0) -> (x*y=w1406:dbl)
            n882 = Multiply(x=w1407, y=w1406) -> (x*y=w1404:dbl)
            n883 = Scale By Power Of 2(n=-48, x=w1404) -> (x*2^n=w1403:dbl)
            n884 = Divide(x=w1403, y=1000000.0) -> (x/y=w1400:dbl)
            n885 = property on="BD 1 Frequency 1 (MHz)" class="DigNum (strict)"("Val(Sgnl)"=w1400) -> ()  [unwired: 2 in, 2 out]
          }
        }
      }
      event "Continuous AOD Scanning": Value Change {
        n886 = event-data() -> ()  [unwired: 7 out]
        n887 = xnode "Read/Write Control"("FPGA VI Reference In"=w1415, "error in"=w1414, "Cont. Scan"="Continuous AOD Scanning") -> ("error out"=w1413:errorcluster)  [unwired: 1 out]
      }
      event "Index": Value Change {
        n888 = event-data() -> ()  [unwired: 7 out]
        n889 = call "Create new save file.vi"("Insert"="", "Ext"=".dat" ("string"), "Index In"="Index") -> ("Path Out"=→"Save file name":path, "Index Out"=w1416:dbl)
        "Save index" <- w1416
        n890 = local write "Index"(w1416) -> ()
      }
      event "AO1", "AO2": Value Change {
        w1431 = 10.0 ("y")
        w1430 = 32767.0 ("y")
        n891 = event-data() -> ()  [unwired: 7 out]
        n892 = local read "AO2"() -> (w1429:dbl)
        n893 = local read "AO1"() -> (w1426:dbl)
        n894 = Multiply(x=w1426, y=w1430) -> (x*y=w1425:dbl)
        n895 = Multiply(x=w1429, y=w1430) -> (x*y=w1428:dbl)
        n896 = Divide(x=w1425, y=w1431) -> (x/y=w1424:dbl)
        n897 = Divide(x=w1428, y=w1431) -> (x/y=w1427:dbl)
        n898 = To Word Integer(number=w1424) -> (16bit integer=w1432:i16)
        n899 = To Word Integer(number=w1427) -> (16bit integer=w1433:i16)
        n900 = xnode "Read/Write Control"("FPGA VI Reference In"=w1423, "error in"=w1422, "AO1 (Y)"=w1432, "AO2 (X)"=w1433) -> ("error out"=w1421:errorcluster)  [unwired: 1 out]
      }
      event "Inject Top:": Value Change {
        n901 = event-data() -> ()  [unwired: 7 out]
        n902 = disable-structure shown="Enabled" {
          disable-tunnel: "Inject Top:" -> [w1435 w1475]
          frame Disabled {
            n903 = local read "Chemyx Syringe Pump Serial Port"() -> (w1436:refnum<visa-resource-name>)
            n904 = local read "Pump write delay (ms)"() -> (w1437:dbl)
            n905 = case shown="True" w1435 {
              tunnel: w1437 -> [w1443 w1457]
              tunnel: w1436 -> [w1440 w1456]
              frame False {
                n906 = flat-sequence {
                  tunnel: w1440 -> [w1444]
                  tunnel: [w1444] -> w1441
                  tunnel: w1443 -> [_]
                  tunnel: [w1447] -> w1442
                  tunnel: w1441 -> [w1447]
                  tunnel: w1442 -> [w1448]
                  tunnel: [w1448] -> w1438
                  tunnel: [w1450] -> w1439
                  tunnel: w1438 -> [w1450]
                  tunnel: w1439 -> [w1452]
                  frame #0 {
                    n907 = call "Write to pump.vi"("string"="enter pump1", "VISA resource name"=w1444) -> ()  [unwired: 1 out]
                  }
                  frame #1 {
                    n908 = Wait (ms)(milliseconds to wait="Pump pause delay (ms)") -> ()  [unwired: 1 out]
                  }
                  frame #2 {
                    n909 = call "Write to pump.vi"("string"="stop", "VISA resource name"=w1448) -> ()  [unwired: 1 out]
                  }
                  frame #3 {
                    n910 = Wait (ms)(milliseconds to wait=u32 500) -> ()  [unwired: 1 out]
                  }
                  frame #4 {
                    n911 = call "Write to pump.vi"("string"="stop", "VISA resource name"=w1452) -> ()  [unwired: 1 out]
                  }
                }
              }
              frame True {
                n912 = flat-sequence {
                  tunnel: w1456 -> [w1466]
                  tunnel: w1457 -> [w1461]
                  tunnel: w1457 -> [w1468]
                  tunnel: w1456 -> [w1469]
                  tunnel: [w1469] -> w1454
                  tunnel: [w1471] -> w1455
                  tunnel: w1454 -> [w1471]
                  tunnel: w1455 -> [w1473]
                  frame #0 {
                    n913 = local read "All Pump Parameters"() -> (w1460:T6)
                    n914 = Unbundle By Name(w1460) -> ("Pump 1"=w1467:T33)
                    n915 = call "Set pump parameters.vi"("Pump write delay (ms)"=w1461, "Volume (uL)"="Ch 2 Inject Volume (uL)", "Rate (uL/h)"="Ch 1 Inject Rate (ul/h)", "Units"=4.0, "Pump #"=1.0, "Pump Parameters In"=w1467, "VISA resource name"=w1466) -> ("Pump Parameters Out"=w1459:T33)  [unwired: 3 in]
                    n916 = Bundle By Name(cluster=w1460, "Pump 1"=w1459) -> (w1458:T6)
                    n917 = local write "All Pump Parameters"(w1458) -> ()
                  }
                  frame #1 {
                    n918 = Wait (ms)(milliseconds to wait=w1468) -> ()  [unwired: 1 out]
                  }
                  frame #2 {
                    n919 = call "Write to pump.vi"("string"="start", "VISA resource name"=w1469) -> ()  [unwired: 1 out]
                  }
                  frame #3 {
                    n920 = Wait (ms)(milliseconds to wait=u32 500) -> ()  [unwired: 1 out]
                  }
                  frame #4 {
                    n921 = call "Write to pump.vi"("string"="start", "VISA resource name"=w1473) -> ()  [unwired: 1 out]
                  }
                }
              }
            }
          }
          frame Enabled {
            n922 = call "hamilton_controller.vi"("Open?"=w1475, "valve"=enum16{"A", "B", "C", "D", "ALL"}."B", "action"=T21."MOVE VALVE") -> ()  [unwired: 8 in, 1 out]
          }
        }
      }
      event "Main:": Value Change {
        n923 = event-data() -> ()  [unwired: 7 out]
        n924 = disable-structure shown="Disabled" {
          disable-tunnel: "Main:" -> [_ w1519]
          frame Disabled {
            n925 = local read "Pump write delay (ms)"() -> (w1480:dbl)
            n926 = case shown="False" w1481 {
              tunnel: w1480 -> [w1487 w1501]
              tunnel: "Chemyx Syringe Pump Serial Port" -> [w1484 w1500]
              frame False {
                n927 = flat-sequence {
                  tunnel: w1484 -> [w1488]
                  tunnel: [w1488] -> w1485
                  tunnel: w1487 -> [_]
                  tunnel: [w1491] -> w1486
                  tunnel: w1485 -> [w1491]
                  tunnel: w1486 -> [w1492]
                  tunnel: [w1492] -> w1482
                  tunnel: [w1494] -> w1483
                  tunnel: w1482 -> [w1494]
                  tunnel: w1483 -> [w1496]
                  frame #0 {
                    n928 = call "Write to pump.vi"("string"="enter pump3", "VISA resource name"=w1488) -> ()  [unwired: 1 out]
                  }
                  frame #1 {
                    n929 = local read "Pump pause delay (ms)"() -> (w1490:u32)
                    n930 = Wait (ms)(milliseconds to wait=w1490) -> ()  [unwired: 1 out]
                  }
                  frame #2 {
                    n931 = call "Write to pump.vi"("string"="stop", "VISA resource name"=w1492) -> ()  [unwired: 1 out]
                  }
                  frame #3 {
                    n932 = Wait (ms)(milliseconds to wait=u32 0) -> ()  [unwired: 1 out]
                  }
                  frame #4 {
                    n933 = call "Write to pump.vi"("string"="stop", "VISA resource name"=w1496) -> ()  [unwired: 1 out]
                  }
                }
              }
              frame True {
                n934 = flat-sequence {
                  tunnel: w1500 -> [w1510]
                  tunnel: w1501 -> [w1505]
                  tunnel: w1501 -> [w1512]
                  tunnel: w1500 -> [w1513]
                  tunnel: [w1513] -> w1498
                  tunnel: [w1516] -> w1499
                  tunnel: w1498 -> [w1516]
                  tunnel: w1499 -> [w1517]
                  frame #0 {
                    n935 = local read "All Pump Parameters"() -> (w1504:T6)
                    n936 = Unbundle By Name(w1504) -> ("Pump 3"=w1511:T33)
                    n937 = call "Set pump parameters.vi"("Pump write delay (ms)"=w1505, "Volume (uL)"="Ch 3 Inject Volume (uL)", "Rate (uL/h)"="Ch 3 Inject Rate (ul/h)", "Units"=4.0, "Pump #"=3.0, "Pump Parameters In"=w1511, "VISA resource name"=w1510) -> ("Pump Parameters Out"=w1503:T33)  [unwired: 3 in]
                    n938 = Bundle By Name(cluster=w1504, "Pump 3"=w1503) -> (w1502:T6)
                    n939 = local write "All Pump Parameters"(w1502) -> ()
                  }
                  frame #1 {
                    n940 = Wait (ms)(milliseconds to wait=w1512) -> ()  [unwired: 1 out]
                  }
                  frame #2 {
                    n941 = call "Write to pump.vi"("string"="start", "VISA resource name"=w1513) -> ()  [unwired: 1 out]
                  }
                  frame #3 {
                    n942 = Wait (ms)(milliseconds to wait=u32 500) -> ()  [unwired: 1 out]
                  }
                  frame #4 {
                    n943 = call "Write to pump.vi"("string"="start", "VISA resource name"=w1517) -> ()  [unwired: 1 out]
                  }
                }
              }
            }
          }
          frame Enabled {
            n944 = call "hamilton_controller.vi"("Open?"=w1519, "valve"=enum16{"A", "B", "C", "D", "ALL"}."A", "action"=T21."MOVE VALVE") -> ()  [unwired: 8 in, 1 out]
          }
        }
      }
      event "Inject Valve B": Value Change {
        n945 = event-data() -> ()  [unwired: 7 out]
        n946 = disable-structure shown="Enabled" {
          disable-tunnel: "Inject Valve B" -> [w1523 w1543]
          frame Disabled {
            n947 = local read "Pump write delay (ms)"() -> (w1525:dbl)
            n948 = flat-sequence {
              tunnel: w1524 -> [w1538]
              tunnel: w1525 -> [w1534]
              tunnel: w1523 -> [_]
              tunnel: w1525 -> [w1540]
              tunnel: w1524 -> [w1541]
              frame #0 {
                n949 = local read "All Pump Parameters"() -> (w1533:T6)
                n950 = Multiply(x=60.0, y="Flush Center Ch Rate (ul/m)") -> (x*y=w1530:dbl)
